vi "StartSequenceAcquisition.vi"(0 "Camera in":refnum<class "Camera.lvclass">, 5 "Exposure":i32=100, 7 "Frames":i32=100, 9 "Interval":i32=100, 11 "error in (no error)":errorcluster) -> (4 "Camera out":refnum<class "Camera.lvclass">, 15 "error out":errorcluster)   [LabVIEW 2020, in "Camera.lvlib" / "Camera.lvclass"]
uses:
  Camera.lvclass
  Camera.lvclass/Camera.ctl
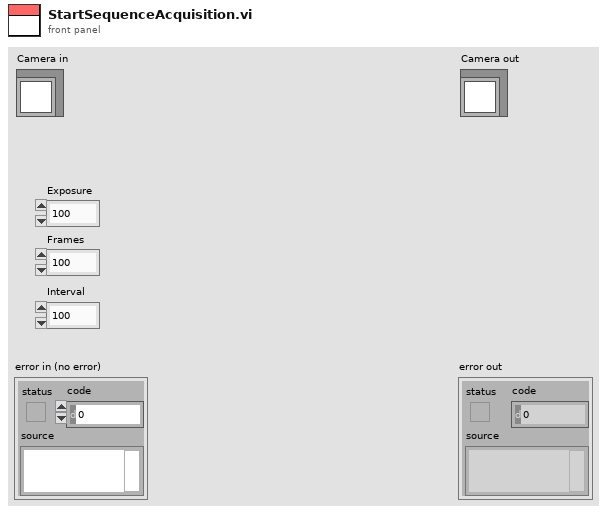
[diagram p1: front panel]
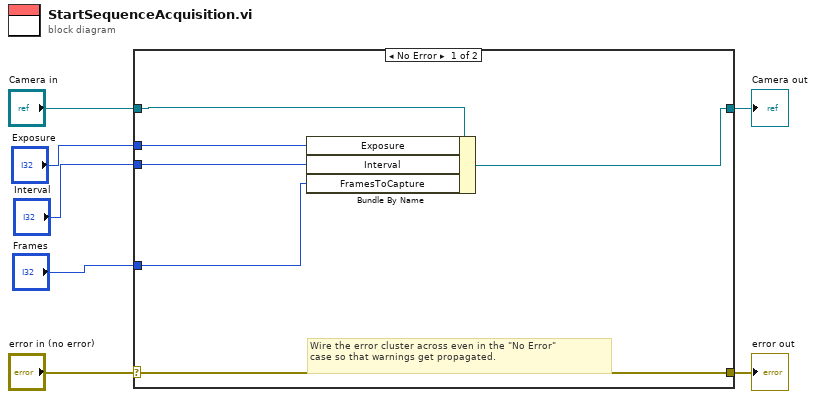
[diagram p0: block diagram]
diagram:
  n1 = case shown="No Error" "error in (no error)" {
    selector: "error in (no error)" -> [w13 w15]
    tunnel: [w13 w15] -> w6
    tunnel: [w11 w14] -> w4
    tunnel: "Camera in" -> [w12 w14]
    tunnel: "Exposure" -> [w10 _]
    tunnel: "Interval" -> [w9 _]
    tunnel: "Frames" -> [w8 _]
    frame No Error {
      # "Wire the error cluster across even in the \"No Error\"\ncase so that warnings get propagated."
      n2 = Bundle By Name(cluster=w12, "Exposure"=w10, "Interval"=w9, "FramesToCapture"=w8) -> (w11:refnum<class "Camera.lvclass">)
    }
    frame Error {
    }
  }
  "error out" <- w6
  "Camera out" <- w4
